vi "onTestSlippage.vi"(7 "Project in":refnum<class "Project.lvclass">, 10 "Properties.Test":refnum<class "Properties.Test.lvclass">) -> (0 "error out":errorcluster, 2 "Properties.Test out":refnum<class "Properties.Test.lvclass">)   [LabVIEW 2021, in "Bananas.lvlib" / "Project.lvclass"]
uses:
  Project.lvclass
  <vilib>/addons/_JKI Toolkits/Caraya/classes/Properties.Test/Properties.Test.lvclass
  C:/Program Files (x86)/National Instruments/LabVIEW 2021/vi.lib/addons/_JKI Toolkits/Caraya/classes/Properties/Properties.lvclass
  Project.lvclass/Project.ctl
  <vilib>/addons/_JKI Toolkits/Caraya/classes/Properties/Properties.lvclass
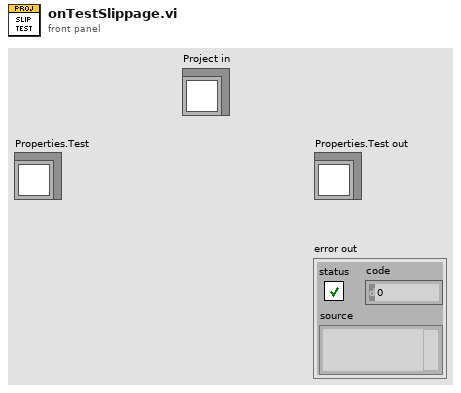
[diagram p1: front panel]
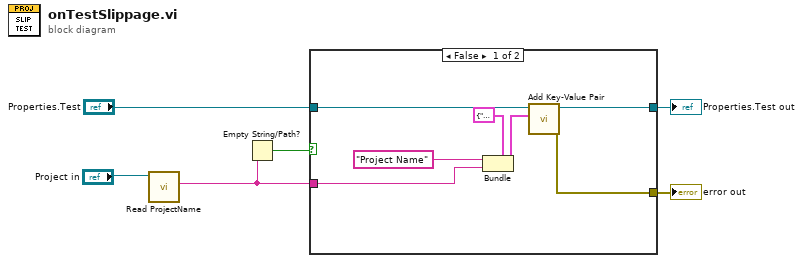
[diagram p0: block diagram]
diagram:
  n1 = call "Read ProjectName.vi"("Project in"="Project in") -> ("ProjectName"=w1:string)  [unwired: 9 in, 1 out]
  n2 = Empty String/Path?(string/path=w1) -> (empty?=w6:bool)
  n3 = case shown="False" w6 {
    tunnel: "Properties.Test" -> [w13 w14]
    tunnel: [w12 w14] -> w4
    tunnel: [w8 _] -> w3
    tunnel: w1 -> [w7 _]
    frame False {
      n4 = Bundle(cluster=cluster{"key":string, "value":variant} {"key"="", "value"=variant} ("entry"), "key"="Project Name", "value"=w7) -> (w10:cluster{"key":string, "value":variant})
      n5 = call <vilib>:"Add Key-Value Pair.vi"("entry"=w10, "Properties in"=w13) -> ("error out"=w8:errorcluster, "Properties out"=w12:refnum<class "Properties.Test.lvclass">)  [unwired: 8 in]
    }
    frame True {
    }
  }
  "error out" <- w3
  "Properties.Test out" <- w4
